vi "Frontview.vi"(0 "Measurement names array":string[](array[string]), 1 "Measurement Values input":dbl[](array[numeric]), 3 "error in (no error)":errorcluster) -> (7 "Measurement values output":dbl[](array[numeric]), 10 "error out":errorcluster)   [LabVIEW 2019, in "Algorithm.lvclass"]
uses:
  FrameworkOverrides/Algorithm.lvclass
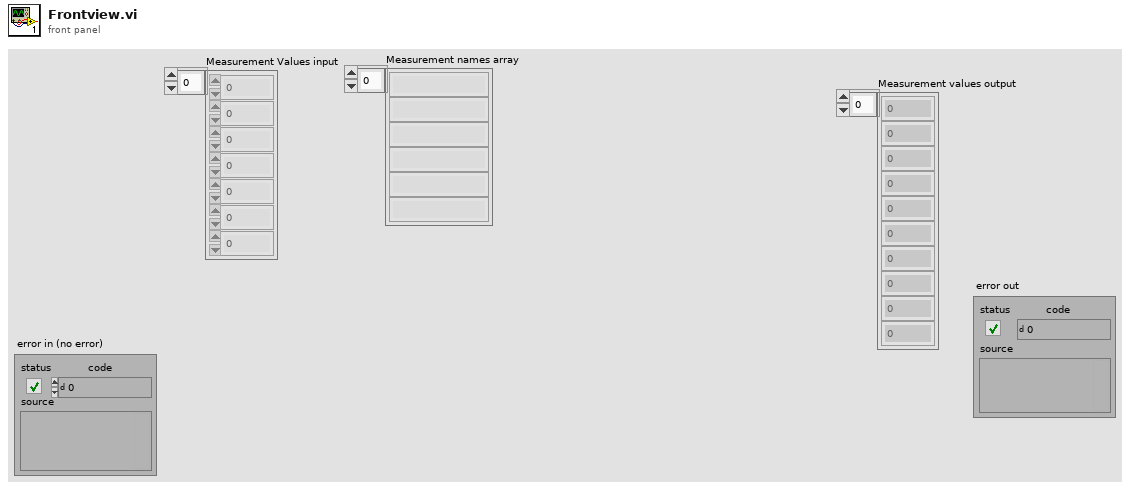
[diagram p1: front panel]
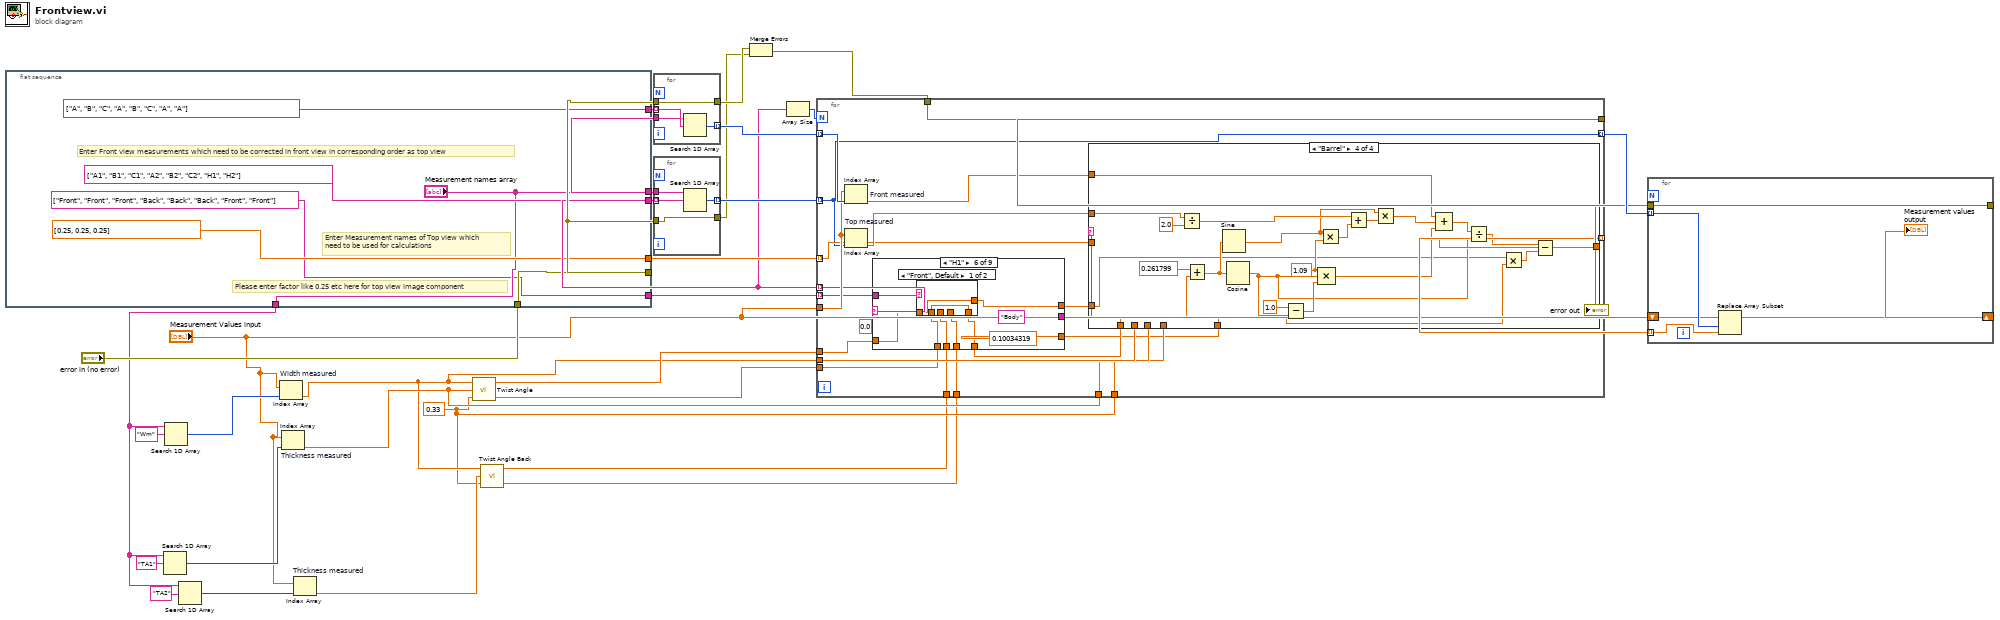
[diagram p0: block diagram]
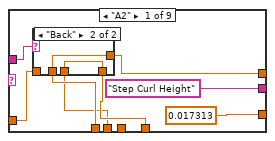
[diagram p2: hidden frame]
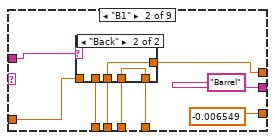
[diagram p4: hidden frame]
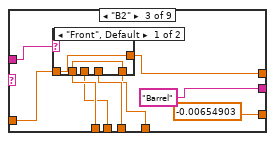
[diagram p6: hidden frame]
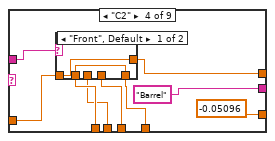
[diagram p8: hidden frame]
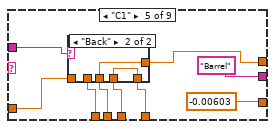
[diagram p10: hidden frame]
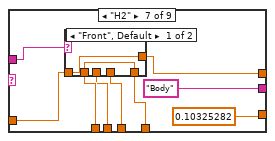
[diagram p13: hidden frame]
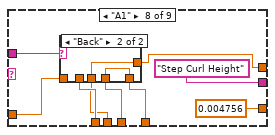
[diagram p15: hidden frame]
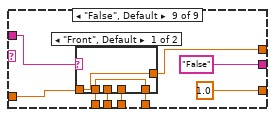
[diagram p17: hidden frame]
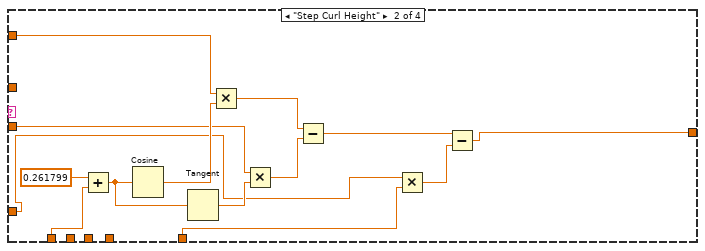
[diagram p20: hidden frame]
diagram:
  w7 = 0.33 ("SideNeck")
  n1 = flat-sequence {
    tunnel: [string[] ["A", "B", "C", "A", "B", "C", "A", "A"] ("To be corrected array")] -> w34
    tunnel: [string[] ["A1", "B1", "C1", "A2", "B2", "C2", "H1", "H2"] ("Top View measurement names array")] -> w2
    tunnel: ["Measurement names array"] -> w33
    tunnel: [dbl[] [0.25, 0.25, 0.25] ("Factor for Top view")] -> w30
    tunnel: [w38] -> w27
    tunnel: "error in (no error)" -> [w38]
    tunnel: ["Measurement names array"] -> w10
    tunnel: [string[] ["Front", "Front", "Front", "Back", "Back", "Back", "Front", "Front"] ("Top View measurement names array")] -> w1
    frame #0 {
      # "Please enter factor like 0.25 etc here for top view image component"
      # "Enter Measurement names of Top view which\nneed to be used for calculations"
      # "Enter Front view measurements which need to be corrected in front view in corresponding order as top view"
    }
  }
  n2 = Search 1D Array(1D array=w10, element="TA1") -> (index of element=w18:i32)  [unwired: 1 in]
  n3 = Search 1D Array(1D array=w10, element="Wm") -> (index of element=w19:i32)  [unwired: 1 in]
  n4 = Search 1D Array(1D array=w10, element="TA2") -> (index of element=w11:i32)  [unwired: 1 in]
  n5 = Index Array "Width measured"(array="Measurement Values input", index=w19) -> (element=w13:dbl)
  n6 = Index Array "Thickness measured"(array="Measurement Values input", index=w18) -> (element=w16:dbl)
  n7 = Index Array "Thickness measured"(array="Measurement Values input", index=w11) -> (element=w8:dbl)
  n8 = call "Twist Angle.vi"("Thickness"=w7, "Thickness Measured"=w16, "Width"=w13) -> ("Theta t (Degree)"=w6:dbl, "Theta t"=w17:dbl)  [unwired: 1 out]
  n9 = call "Twist Angle Back.vi"("Thickness"=w7, "Thickness Measured"=w8, "Width"=w13) -> ("Theta t (Degree)"=w4:dbl, "Theta t"=w5:dbl)  [unwired: 1 out]
  n10 = for {
    tunnel: w34 -> [w44] mode=indexing
    tunnel: w33 -> [w43]
    tunnel: [w42] -> w31 mode=indexing
    tunnel: w27 -> [w41]
    tunnel: [w41] -> w26
    n11 = Search 1D Array(1D array=w43, element=w44) -> (index of element=w42:i32)  [unwired: 1 in]
  }
  n12 = for {
    tunnel: [w48] -> w32 mode=indexing
    tunnel: w2 -> [w47] mode=indexing
    tunnel: w33 -> [w46]
    tunnel: w27 -> [w45]
    tunnel: [w45] -> w25
    n13 = Search 1D Array(1D array=w46, element=w47) -> (index of element=w48:i32)  [unwired: 1 in]
  }
  n14 = Merge Errors(w26, w25) -> (w24:errorcluster)
  n15 = Array Size(array=w2) -> (size(s)=w3:i32)
  n16 = for {
    N: w3 -> [_]
    tunnel: w32 -> [w50] mode=indexing
    tunnel: w31 -> [w69] mode=indexing
    tunnel: w30 -> [w59] mode=indexing
    tunnel: [w50] -> w29 mode=indexing
    tunnel: "Measurement Values input" -> [w68]
    tunnel: w24 -> [w67]
    tunnel: [w67] -> w23
    tunnel: w17 -> [w57]
    tunnel: w6 -> [w56]
    tunnel: [w58] -> w14 mode=indexing
    tunnel: w2 -> [w66] mode=indexing
    tunnel: w13 -> [w62]
    tunnel: w16 -> [w61]
    tunnel: w7 -> [w60]
    tunnel: w5 -> [w55]
    tunnel: w4 -> [w54]
    tunnel: w1 -> [w49] mode=indexing
    (unwired) 0.0 ("Factor for Top view")
    n17 = Index Array "Front measured"(array=w68, index=w69) -> (element=w64:dbl)
    n18 = Index Array "Top measured"(array=w68, index=w50) -> (element=w63:dbl)
    n19 = case shown="\"H1\"" w66 {
      tunnel: ["Step Curl Height" "Barrel" "Barrel" "Barrel" "Barrel" "Body" "Body" "Step Curl Height" "False"] -> w65
      tunnel: [0.017313 ("Factor for Top view") -0.006549 ("Factor for Top view") -0.00654903 ("Factor for Top view") -0.05096 ("Factor for Top view") -0.00603 ("Factor for Top view") 0.10034319 ("Factor for Top view") 0.10325282 ("Factor for Top view") 0.004756 ("Factor for Top view") 1.0 ("Factor for Top view")] -> w51
      tunnel: w57 -> [w73 w88 w101 w114 w127 w140 w153 w166 w179]
      tunnel: w56 -> [w72 w87 w100 w113 w126 w139 w152 w165 w178]
      tunnel: w55 -> [w71 w86 w99 w112 w125 w138 w151 w164 w177]
      tunnel: w54 -> [_ w85 w98 w111 w124 w137 w150 w163 w176]
      tunnel: [w75 w83 w96 w110 w122 w135 w148 w161 w175] -> w53
      tunnel: [w74 w84 w97 w109 w123 w136 w149 w162 w174] -> w52
      tunnel: w49 -> [w70 w82 w95 w108 w121 w134 w147 w160 w173]
      frame "A2" {
        n20 = case shown="\"Back\"" w70 {
          tunnel: w73 -> [w79 _]
          tunnel: w72 -> [w78 w81]
          tunnel: w71 -> [_ w80]
          tunnel: [w79 w81] -> w75
          tunnel: [w78 w80] -> w74
          frame "Front", Default {
          }
          frame "Back" {
          }
        }
      }
      frame "B1" {
        n21 = case shown="\"Back\"" w82 {
          tunnel: w88 -> [w92 _]
          tunnel: w87 -> [w91 _]
          tunnel: w86 -> [_ w94]
          tunnel: w85 -> [_ w93]
          tunnel: [w92 w94] -> w83
          tunnel: [w91 w93] -> w84
          frame "Front", Default {
          }
          frame "Back" {
          }
        }
      }
      frame "B2" {
        n22 = case shown="\"Front\", Default" w95 {
          tunnel: w101 -> [w105 _]
          tunnel: w100 -> [w104 _]
          tunnel: w99 -> [_ w107]
          tunnel: w98 -> [_ w106]
          tunnel: [w105 w107] -> w96
          tunnel: [w104 w106] -> w97
          frame "Front", Default {
          }
          frame "Back" {
          }
        }
      }
      frame "C2" {
        n23 = case shown="\"Front\", Default" w108 {
          tunnel: w114 -> [w118 _]
          tunnel: w113 -> [w117 _]
          tunnel: w112 -> [_ w120]
          tunnel: w111 -> [_ w119]
          tunnel: [w118 w120] -> w110
          tunnel: [w117 w119] -> w109
          frame "Front", Default {
          }
          frame "Back" {
          }
        }
      }
      frame "C1" {
        n24 = case shown="\"Back\"" w121 {
          tunnel: w127 -> [w131 _]
          tunnel: w126 -> [w130 _]
          tunnel: w125 -> [_ w133]
          tunnel: w124 -> [_ w132]
          tunnel: [w131 w133] -> w122
          tunnel: [w130 w132] -> w123
          frame "Front", Default {
          }
          frame "Back" {
          }
        }
      }
      frame "H1" {
        n25 = case shown="\"Front\", Default" w134 {
          tunnel: w140 -> [w144 _]
          tunnel: w139 -> [w143 _]
          tunnel: w138 -> [_ w146]
          tunnel: w137 -> [_ w145]
          tunnel: [w144 w146] -> w135
          tunnel: [w143 w145] -> w136
          frame "Front", Default {
          }
          frame "Back" {
          }
        }
      }
      frame "H2" {
        n26 = case shown="\"Front\", Default" w147 {
          tunnel: w153 -> [w157 _]
          tunnel: w152 -> [w156 _]
          tunnel: w151 -> [_ w159]
          tunnel: w150 -> [_ w158]
          tunnel: [w157 w159] -> w148
          tunnel: [w156 w158] -> w149
          frame "Front", Default {
          }
          frame "Back" {
          }
        }
      }
      frame "A1" {
        n27 = case shown="\"Back\"" w160 {
          tunnel: w166 -> [w170 _]
          tunnel: w165 -> [w169 _]
          tunnel: w164 -> [_ w172]
          tunnel: w163 -> [_ w171]
          tunnel: [w170 w172] -> w161
          tunnel: [w169 w171] -> w162
          frame "Front", Default {
          }
          frame "Back" {
          }
        }
      }
      frame "False", Default {
        n28 = case shown="\"Front\", Default" w173 {
          tunnel: w179 -> [w183 _]
          tunnel: w178 -> [w182 _]
          tunnel: w177 -> [_ w185]
          tunnel: w176 -> [_ w184]
          tunnel: [w183 w185] -> w175
          tunnel: [w182 w184] -> w174
          frame "Front", Default {
          }
          frame "Back" {
          }
        }
      }
    }
    n29 = case shown="\"Barrel\"" w65 {
      tunnel: w64 -> [w186 w191 _ w220]
      tunnel: w63 -> [_ _ w211 w234]
      tunnel: w52 -> [_ w200 w217 w238]
      tunnel: w62 -> [_ _ _ _]
      tunnel: w61 -> [_ _ _ _]
      tunnel: w60 -> [_ _ _ _]
      tunnel: w59 -> [_ w194 _ _]
      tunnel: [w186 w188 w202 w219] -> w58
      tunnel: w53 -> [_ w189 w204 w222]
      tunnel: w51 -> [_ w190 w205 w223]
      frame "False", Default {
      }
      frame "Step Curl Height" {
        n30 = Add(x=0.261799, y=w200) -> (x+y=w197:dbl)
        n31 = Cosine(x=w197) -> (cos(x)=w198:dbl)
        n32 = Tangent(1:w197) -> (0:w196:dbl)
        n33 = Multiply(x=w191, y=w198) -> (x*y=w193:dbl)
        n34 = Multiply(x=w194, y=w196) -> (x*y=w195:dbl)
        n35 = Subtract(x=w193, y=w195) -> (x-y=w187:dbl)
        n36 = Multiply(x=w189, y=w190) -> (x*y=w192:dbl)
        n37 = Subtract(x=w187, y=w192) -> (x-y=w188:dbl)
      }
      frame "Body" {
        n38 = Add(x=0.261799, y=w217) -> (x+y=w215:dbl)
        n39 = Subtract(x=w211, y=0.9) -> (x-y=w213:dbl)
        n40 = Sine & Cosine(0:w215) -> (1:w206:dbl, 2:w208:dbl)
        n41 = Multiply(x=0.25, y=w213) -> (x*y=w209:dbl)
        n42 = Multiply(x=w209, y=w208) -> (x*y=w210:dbl)
        n43 = Subtract(x=w211, y=w210) -> (x-y=w207:dbl)
        n44 = Multiply(x=w207, y=w206) -> (x*y=w201:dbl)
        n45 = Multiply(x=w204, y=w205) -> (x*y=w203:dbl)
        n46 = Subtract(x=w201, y=w203) -> (x-y=w202:dbl)
      }
      frame "Barrel" {
        w232 = 1.09 ("value")
        n47 = Divide(x=w234, y=2.0) -> (x/y=w230:dbl)
        n48 = Add(x=0.261799, y=w238) -> (x+y=w235:dbl)
        n49 = Sine(x=w235) -> (sin(x)=w228:dbl)
        n50 = Cosine(x=w235) -> (cos(x)=w224:dbl)
        n51 = Subtract(x=1.0, y=w224) -> (x-y=w236:dbl)
        n52 = Compound Arithmetic op=MULTIPLY(w232, w224, w236) -> (w227:dbl)
        n53 = Multiply(x=w228, y=w232) -> (x*y=w231:dbl)
        n54 = Add(x=w230, y=w231) -> (x+y=w229:dbl)
        n55 = Multiply(x=w228, y=w229) -> (x*y=w226:dbl)
        n56 = Compound Arithmetic op=ADD(w220, w226, w227) -> (w225:dbl)
        n57 = Divide(x=w225, y=w224) -> (x/y=w218:dbl)
        n58 = Multiply(x=w222, y=w223) -> (x*y=w221:dbl)
        n59 = Subtract(x=w218, y=w221) -> (x-y=w219:dbl)
      }
    }
  }
  n60 = for {
    tunnel: w29 -> [w244] mode=indexing
    shift-right: [w243] -> w15
    shift-left: "Measurement Values input" -> [w242]
    tunnel: w23 -> [w241]
    tunnel: [w241] -> w22
    tunnel: w14 -> [w240] mode=indexing
    n61 = Replace Array Subset(array=w242, new element=w240, index=w244) -> (w243:dbl[])
  }
  "error out" <- w22
  "Measurement values output" <- w15
